vi "Associated Research 78XX Series Creating and Saving a File.vi"(8 "error in (no error)":errorcluster, 11 "VISA resource name":refnum<visa-resource-name>="COM1") -> (0 "error out":errorcluster)   [LabVIEW 2020]
doc: "This VI is an example on how to Create and Save files in the ARI-78XX (HiPOT Ultra) series.\n\nIt will create a file called \"RandomT\" and fill it with default ACW, DCW, IR test types."
uses:
  <instrlib>/Associated Research 78XX Series/Public/Configure/Steps/Low Level/Scanner Settings.ctl
  <instrlib>/Associated Research 78XX Series/Public/Configure/Steps/Low Level/ACW Test Parameters.ctl
  <instrlib>/Associated Research 78XX Series/Public/Configure/Steps/Low Level/DCW Test Parameters.ctl
  <instrlib>/Associated Research 78XX Series/Public/Configure/Steps/Low Level/IR Test Parameters.ctl
  <instrlib>/Associated Research 78XX Series/Public/Configure/Steps/Low Level/GND Test Parameters.ctl
  <instrlib>/Associated Research 78XX Series/Associated Research 78XX Series.lvlib
panel:
  in  "Scanner Channel (0 - 16) (0)":u32
  in  "GND Test Paramameters":T1={"Current (1 - 32 A) (25A)"=25.0, "Voltage (3 - 8 V) (8V)"=8.0, "High Limit (0 - 200 mohm)(100 mohm)"=100, "Low Limit (0 - 200 mohm)(0 mohm)"=0, "High Limit V (0 - 6.00 V) (6V)"=6.0, "Low Limit V (0 - 6.00 V) (0V)"=0.0, "Dwell Time (0.0, 0.5 - 999.9 s) (1.0S)"=1.0, "Offset (0 - 200 mohm) (0mohm)"=0, "Offset V (0 - 6.00 V) (0V)"=0.0, "Frequency (50/60 HZ) (50HZ)"=enum."50", "Auto Offset (F: Off)"=FALSE} {"Offset V (0 - 6.00 V) (0V)" format="%#.2f"; "Dwell Time (0.0, 0.5 - 999.9 s) (1.0S)" format="%.1f"; "Low Limit V (0 - 6.00 V) (0V)" format="%#.2f"; "High Limit V (0 - 6.00 V) (6V)" format="%#.2f"; "Voltage (3 - 8 V) (8V)" format="%.2f"; "Current (1 - 32 A) (25A)" format="%.2f"}
  in  "File Name":string="RandomT"
  in  "IR Test Parameters":T2={"Voltage (1000)"=1000, "High Limit(0.0, 0.5 - 50000 Megohms) (5)"=0.0, "Low Limit(0.1 - 50000 Megohms) (0)"=0.1, "Ramp Up Time (0.1 - 999.9 seconds) (0.1)"=0.1, "Delay Time (0.0, 1.0 - 999.9 seconds) (0.5)"=0.5, "Ramp Down Time (0.0 - 999.9 seconds) (0) "=0.0, "Charge LO (0)"=0.0, "Auto Charge LO (F: Off)"=FALSE, "Dwell Time (0.0, 1.0 - 999.9 seconds) (0.5)"=0.5} {"Dwell Time (0.0, 1.0 - 999.9 seconds) (0.5)" format="%.1f"; "Ramp Down Time (0.0 - 999.9 seconds) (0)" format="%.1f"; "Charge LO (0)" format="%.2f"; "Delay Time (0.0, 1.0 - 999.9 seconds) (0.5)" format="%.1f"; "Ramp Up Time (0.1 - 999.9 seconds) (0.1)" format="%.1f"; "Low Limit(0.1 - 50000 Megohms) (0)" format="%.1f"; "High Limit(0.0, 0.5 - 50000 Megohms) (5)" format="%.1f"}
  in  "DCW Test Parameters":T3={"Voltage (1500)"=1500, "High Limit(0.0 - 10,000 microamps) (10)"=10000.0, "Low Limit(0.0 - 10,000 microamps) (0)"=0.0, "Ramp Up Time (0.4 - 999.9 seconds) (0.4)"=0.4, "Dwell Time (0, 0.4 - 999.9 seconds) (1)"=1.0, "Ramp Down Time (0, 1.0 - 999.9 seconds) (0) "=0.0, "Charge LO (0.0 - 350uA)"=0.0, "Arc Sense (1 - 9) (5)"=5, "Arc Detect (F: Off)"=FALSE, "Continuity (F: Off)"=FALSE, "Auto Charge LO (F: Off)"=FALSE, "Low Range (F: Off)"=FALSE, "Offset (0.0 - 10,000uA)"=0.0, "Ramp-Hi (0.0 - 10,000uA)"=0.0, "Range (F: AUTO)"=enum."AUTO"} {"Ramp-Hi (0.0 - 10,000uA)" format="%.2f"; "Offset (0.0 - 10,000uA)" format="%.2f"; "Ramp Down Time (0, 1.0 - 999.9 seconds) (0)" format="%.1f"; "Charge LO (0.0 - 350uA)" format="%.2f"; "Dwell Time (0, 0.4 - 999.9 seconds) (1)" format="%.1f"; "Ramp Up Time (0.4 - 999.9 seconds) (0.4)" format="%.1f"; "Low Limit(0.0 - 10,000 microamps) (0)" format="%.1f"; "High Limit(0.0 - 10,000 microamps) (10)" format="%.1f"}
  in  "ACW Test Parameters":T4={"Voltage (1240)"=1240, "High Limit Total (10)"=5.0, "Low Limit Total (0)"=0.0, "High Limit Real(10)"=10.0, "Low Limit Real (0)"=0.0, "Ramp Up Time (0.1 - 999.9 seconds) (0.1)"=0.1, "Dwell Time (0, 0.2 - 999.9 seconds) (1)"=1.0, "Ramp Down Time (0.0 - 999.9 seconds) (1)"=0.0, "Arc Sense (1 - 9) (5)"=5, "Arc Detect (F: Off)"=FALSE, "Continuity (F: Off)"=FALSE, "Range  "=enum."AUTO", "Offset (0)"=0.0, "Auto Offset (F: Off)"=FALSE, "Frequency"=enum."60"} {"Offset (0)" format="%.2f"; "Ramp Down Time (0.0 - 999.9 seconds) (1)" min=0.0 max=999.9 step=0.1 format="%.1f"; "Low Limit Real (0)" min=0.0 max=999.9 step=0.001 format="%.3f"; "High Limit Real(10)" min=0.0 max=100.0 format="%.2f"; "Arc Sense (1 - 9) (5)" min=1 max=9; "Dwell Time (0, 0.2 - 999.9 seconds) (1)" min=0.0 max=999.9 step=0.1 format="%.1f"; "Ramp Up Time (0.1 - 999.9 seconds) (0.1)" min=0.1 max=999.9 step=0.1 format="%.1f"; "Low Limit Total (0)" min=0.0 max=999.9 step=0.001 format="%.3f"; "High Limit Total (10)" min=0.0 max=100.0 format="%.2f"; "Voltage (1240)" min=0 max=12000}
  in  "Internal Scanner Exists?":bool
  in  "Scanner Settings":T5={"Scan1"=1, "Scan2"=1, "Scan3"=1, "Scan4"=1, "Scan5"=1, "Scan6"=1, "Scan7"=1, "Scan8"=1, "Scan9"=1, "Scan10"=1, "Scan11"=1, "Scan12"=1, "Scan13"=1, "Scan14"=1, "Scan15"=1, "Scan16"=1} {"Scan16" scale=0.0..2.0; "Scan15" scale=0.0..2.0; "Scan14" scale=0.0..2.0; "Scan13" scale=0.0..2.0; "Scan12" scale=0.0..2.0; "Scan11" scale=0.0..2.0; "Scan10" scale=0.0..2.0; "Scan9" scale=0.0..2.0; "Scan8" scale=0.0..2.0; "Scan7" scale=0.0..2.0; "Scan6" scale=0.0..2.0; "Scan5" scale=0.0..2.0; "Scan4" scale=0.0..2.0; "Scan3" min=0 max=2 scale=0.0..2.0; "Scan2" min=0 max=2 scale=0.0..2.0; "Scan1" min=0 max=2 scale=0.0..2.0}
  out "Error Occured?":bool
  # "On\nOff"
  # "On\nOff"
  # "On\nOff"
  # "On\nOff"
  # "On\nOff"
  # "Fixed\nAuto"
  # "On\nOff"
  # "On\nOff"
  # "On\nOff"
  # "On\nOff"
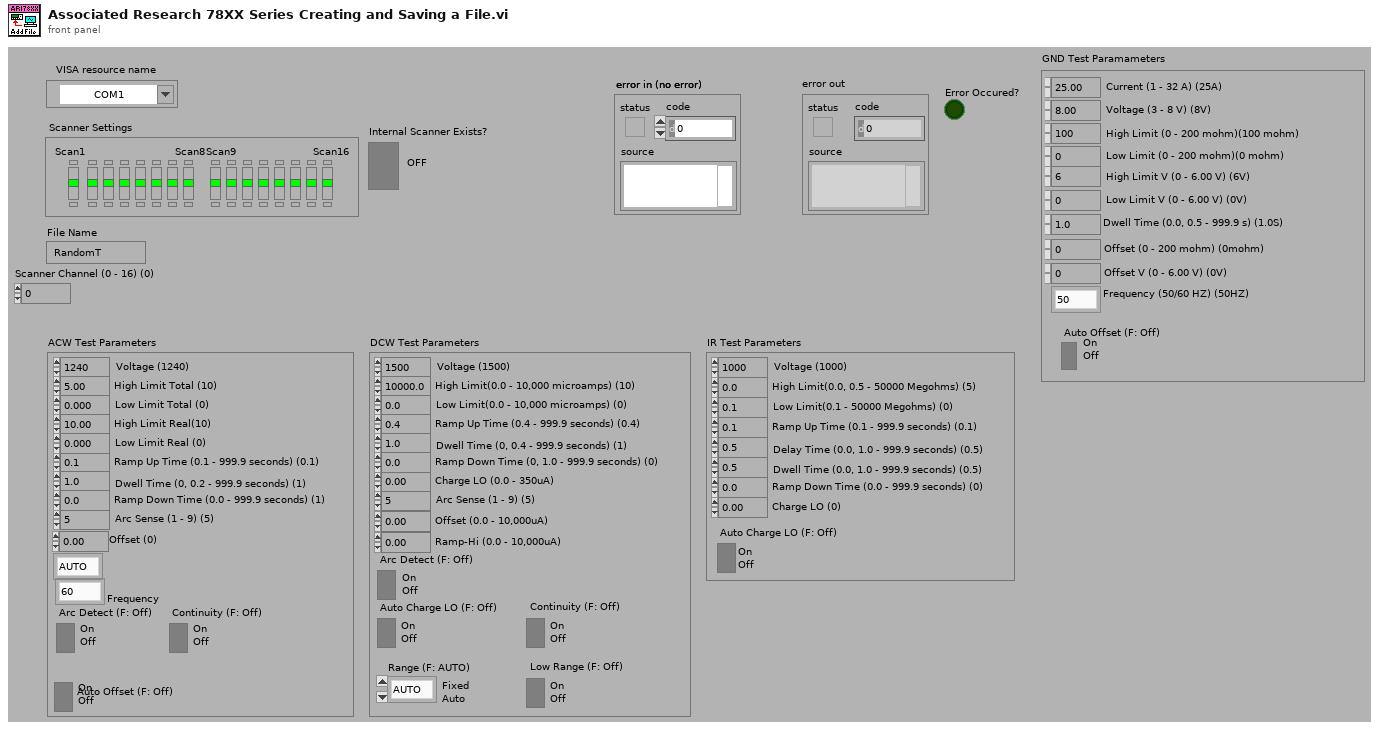
[diagram p1: front panel]
types:
  T1 = typedef "Associated Research 78XX Series.lvlib/GND Test Parameters.ctl" = cluster{"Current (1 - 32 A) (25A)":dbl, "Voltage (3 - 8 V) (8V)":dbl, "High Limit (0 - 200 mohm)(100 mohm)":i32, "Low Limit (0 - 200 mohm)(0 mohm)":i32, "High Limit V (0 - 6.00 V) (6V)":dbl, "Low Limit V (0 - 6.00 V) (0V)":dbl, "Dwell Time (0.0, 0.5 - 999.9 s) (1.0S)":dbl, "Offset (0 - 200 mohm) (0mohm)":i32, "Offset V (0 - 6.00 V) (0V)":dbl, "Frequency (50/60 HZ) (50HZ)":enum16{"50", "60"}, "Auto Offset (F: Off)":bool}
  T2 = typedef "Associated Research 78XX Series.lvlib/IR Test Parameters.ctl" = cluster{"Voltage (1000)":i32, "High Limit(0.0, 0.5 - 50000 Megohms) (5)":dbl, "Low Limit(0.1 - 50000 Megohms) (0)":dbl, "Ramp Up Time (0.1 - 999.9 seconds) (0.1)":dbl, "Delay Time (0.0, 1.0 - 999.9 seconds) (0.5)":dbl, "Ramp Down Time (0.0 - 999.9 seconds) (0) ":dbl, "Charge LO (0)":dbl, "Auto Charge LO (F: Off)":bool, "Dwell Time (0.0, 1.0 - 999.9 seconds) (0.5)":dbl}
  T3 = typedef "Associated Research 78XX Series.lvlib/DCW Test Parameters.ctl" = cluster{"Voltage (1500)":i32, "High Limit(0.0 - 10,000 microamps) (10)":dbl, "Low Limit(0.0 - 10,000 microamps) (0)":dbl, "Ramp Up Time (0.4 - 999.9 seconds) (0.4)":dbl, "Dwell Time (0, 0.4 - 999.9 seconds) (1)":dbl, "Ramp Down Time (0, 1.0 - 999.9 seconds) (0) ":dbl, "Charge LO (0.0 - 350uA)":dbl, "Arc Sense (1 - 9) (5)":i32, "Arc Detect (F: Off)":bool, "Continuity (F: Off)":bool, "Auto Charge LO (F: Off)":bool, "Low Range (F: Off)":bool, "Offset (0.0 - 10,000uA)":dbl, "Ramp-Hi (0.0 - 10,000uA)":dbl, "Range (F: AUTO)":enum16{"AUTO", "FIXED"}}
  T4 = typedef "Associated Research 78XX Series.lvlib/ACW Test Parameters.ctl" = cluster{"Voltage (1240)":i32, "High Limit Total (10)":dbl, "Low Limit Total (0)":dbl, "High Limit Real(10)":dbl, "Low Limit Real (0)":dbl, "Ramp Up Time (0.1 - 999.9 seconds) (0.1)":dbl, "Dwell Time (0, 0.2 - 999.9 seconds) (1)":dbl, "Ramp Down Time (0.0 - 999.9 seconds) (1)":dbl, "Arc Sense (1 - 9) (5)":i32, "Arc Detect (F: Off)":bool, "Continuity (F: Off)":bool, "Range  ":enum16{"AUTO", "FIXED"}, "Offset (0)":dbl, "Auto Offset (F: Off)":bool, "Frequency":enum16{"50", "60", "400", "800"}}
  T5 = typedef "Associated Research 78XX Series.lvlib/Scanner Settings.ctl" = cluster{"Scan1":i32, "Scan2":i32, "Scan3":i32, "Scan4":i32, "Scan5":i32, "Scan6":i32, "Scan7":i32, "Scan8":i32, "Scan9":i32, "Scan10":i32, "Scan11":i32, "Scan12":i32, "Scan13":i32, "Scan14":i32, "Scan15":i32, "Scan16":i32}
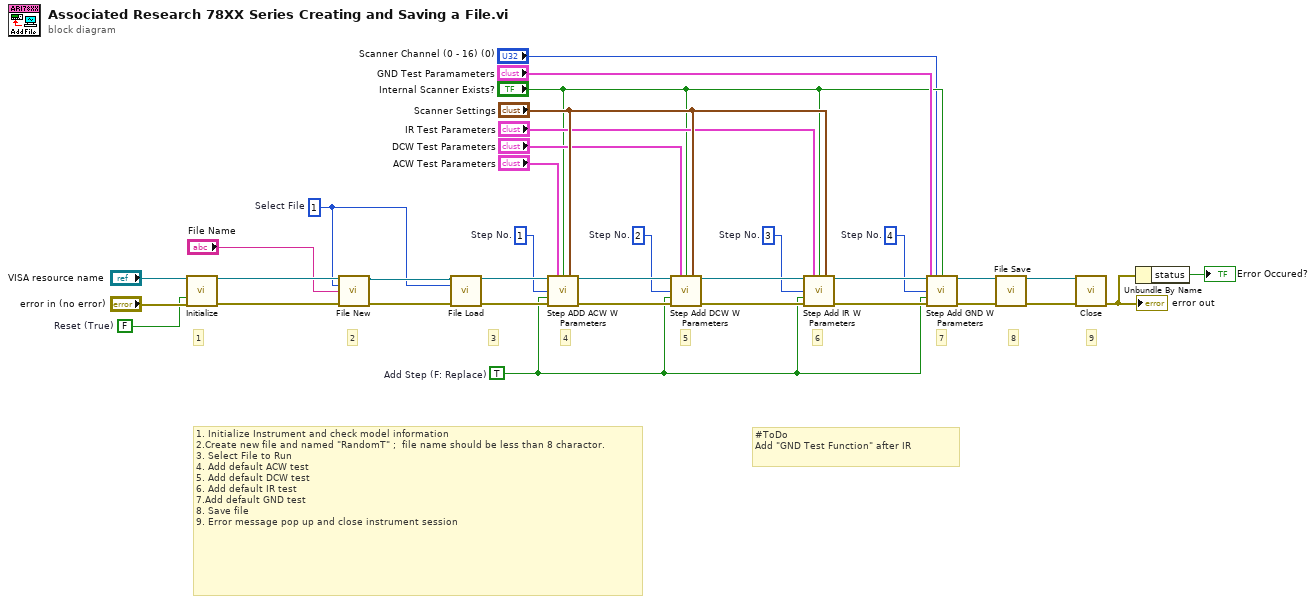
[diagram p0: block diagram]
diagram:
  w5 = 4  # Step No.
  w18 = 3  # Step No.
  w21 = 2  # Step No.
  w24 = 1  # Step No.
  w1 = TRUE  # Add Step (F: Replace)
  w15 = 1  # Select File
  w33 = FALSE  # Reset (True)
  # "9"
  # "#ToDo\nAdd \"GND Test Function\" after IR"
  # "6"
  # "5"
  # "4"
  # "8"
  # "1. Initialize Instrument and check model information\n2.Create new file and named \"RandomT\" ;  file name should be less than 8 charactor.\n3. Select File to Run\n4. Add default ACW test\n5. Add default DCW test\n6. Add default IR test\n7.Add default GND test\n8. Save file\n9. Error message pop up and close instrument session"
  # "7"
  # "3"
  # "2"
  # "1"
  n1 = call <instrlib>:"Initialize.vi"("VISA resource name"="VISA resource name", "Reset (True)"=w33, "error in (no error)"="error in (no error)") -> ("VISA resource name out"=w30:refnum<visa-resource-name>, "error out"=w28:errorcluster)  [unwired: 10 in, 1 out]
  n2 = call <instrlib>:"File New.vi"("VISA resource name"=w30, "File Number (1)"=w15, "File Name"="File Name", "error in (no error)"=w28) -> ("VISA resource name out"=w27:refnum<visa-resource-name>, "error out"=w10:errorcluster)  [unwired: 10 in]
  n3 = call <instrlib>:"File Load.vi"("VISA resource name"=w27, "File Number (1-2000)"=w15, "error in (no error)"=w10) -> ("VISA resource name out"=w26:refnum<visa-resource-name>, "error out"=w25:errorcluster)  [unwired: 11 in]
  n4 = call <instrlib>:"Step ADD ACW W Parameters.vi"("VISA resource name"=w26, "ACW Test Parameters"="ACW Test Parameters", "Internal scanner?"="Internal Scanner Exists?", "Scanner Settings"="Scanner Settings", "Step Selection (1-200)"=w24, "Add Step"=w1, "error in (no error)"=w25) -> ("VISA resource name out"=w23:refnum<visa-resource-name>, "error out"=w22:errorcluster)  [unwired: 7 in]
  n5 = call <instrlib>:"Step Add DCW W Parameters.vi"("VISA resource name"=w23, "DCW Test Parameters (in)"="DCW Test Parameters", "Internal Scanner Exists?"="Internal Scanner Exists?", "Scanner Settings"="Scanner Settings", "Step Selection (1-200)"=w21, "Add Step"=w1, "error in (no error)"=w22) -> ("VISA resource name out"=w20:refnum<visa-resource-name>, "error out"=w19:errorcluster)  [unwired: 7 in]
  n6 = call <instrlib>:"Step Add IR W Parameters.vi"("VISA resource name"=w20, "IR Test Parameters in"="IR Test Parameters", "Internal Scanner Exists?"="Internal Scanner Exists?", "Scanner Settings"="Scanner Settings", "Step Selection (1-200)"=w18, "Add Step"=w1, "error in (no error)"=w19) -> ("VISA resource name out"=w7:refnum<visa-resource-name>, "error out"=w9:errorcluster)  [unwired: 7 in]
  n7 = call <instrlib>:"Step Add GND W Parameters.vi"("VISA resource name"=w7, "Scanner Channel (0 - 16) (0)"="Scanner Channel (0 - 16) (0)", "Internal Scanner Exists?"="Internal Scanner Exists?", "GND Test Paramameters"="GND Test Paramameters", "Step Selection (1-200)"=w5, "Add Step"=w1, "error in (no error)"=w9) -> ("VISA resource name out"=w6:refnum<visa-resource-name>, "error out"=w8:errorcluster)  [unwired: 7 in]
  n8 = call <instrlib>:"File Save.vi"("VISA resource name"=w6, "error in (no error)"=w8) -> ("VISA resource name out"=w17:refnum<visa-resource-name>, "error out"=w16:errorcluster)  [unwired: 12 in]
  n9 = call <instrlib>:"Close.vi"("VISA resource name"=w17, "error in (no error)"=w16) -> ("error out"=w31:errorcluster)  [unwired: 13 in]
  "error out" <- w31
  n10 = Unbundle By Name(w31) -> ("status"=→"Error Occured?":bool)
